vi "helper-snapshot-list.vi"(10 "ADDR":u8=1 min=1 max=99 step=1, 11 "IOnodes in":T1[](array[typedef])=[{"ADDR"=307, "Label"="ACID", "Type"=enum."DO", "Mode"=enum."RIO", "Value"="", "Tags"="", "calibration"=[{"X"=0.0, "Y"=0.0}, {"X"=0.0, "Y"=0.0}]}, {"ADDR"=309, "Label"="ALFA1", "Type"=enum."DO", "Mode"=enum."RIO", "Value"="", "Tags"="", "calibration"=[{"X"=0.0, "Y"=0.0}, {"X"=0.0, "Y"=0.0}]}, {"ADDR"=305, "Label"="BASE", "Type"=enum."DO", "Mode"=enum."RIO", "Value"="", "Tags"="", "calibration"=[{"X"=0.0, "Y"=0.0}, {"X"=0.0, "Y"=0.0}]}, {"ADDR"=311, "Label"="BETA1", "Type"=enum."DO", "Mode"=enum."RIO", "Value"="", "Tags"="", "calibration"=[{"X"=0.0, "Y"=0.0}, {"X"=0.0, "Y"=0.0}]}, {"ADDR"=210, "Label"="CIRCULATORS", "Type"=enum."DO", "Mode"=enum."RIO", "Value"="", "Tags"="", "calibration"=[{"X"=0.0, "Y"=0.0}, {"X"=0.0, "Y"=0.0}]}, {"ADDR"=200, "Label"="CNET", "Type"=enum."DO", "Mode"=enum."RIO", "Value"="", "Tags"="", "calibration"=[{"X"=0.0, "Y"=0.0}, {"X"=0.0, "Y"=0.0}]}, {"ADDR"=201, "Label"="CNETFOG", "Type"=enum."DO", "Mode"=enum."RIO", "Value"="", "Tags"="", "calibration"=[{"X"=0.0, "Y"=0.0}, {"X"=0.0, "Y"=0.0}]}, {"ADDR"=117, "Label"="CO2", "Type"=enum."DO", "Mode"=enum."RIO", "Value"="", "Tags"="", "calibration"=[{"X"=0.0, "Y"=0.0}, {"X"=0.0, "Y"=0.0}]}, {"ADDR"=316, "Label"="COLCHIL", "Type"=enum."DO", "Mode"=enum."RIO", "Value"="", "Tags"="", "calibration"=[{"X"=0.0, "Y"=0.0}, {"X"=0.0, "Y"=0.0}]}, {"ADDR"=112, "Label"="COOLFAN", "Type"=enum."DO", "Mode"=enum."RIO", "Value"="", "Tags"="", "calibration"=[{"X"=0.0, "Y"=0.0}, {"X"=0.0, "Y"=0.0}]}, {"ADDR"=211, "Label"="FECTORY_VENT", "Type"=enum."DO", "Mode"=enum."RIO", "Value"="", "Tags"="", "calibration"=[{"X"=0.0, "Y"=0.0}, {"X"=0.0, "Y"=0.0}]}, {"ADDR"=208, "Label"="H1_CURTAIN", "Type"=enum."DO", "Mode"=enum."RIO", "Value"="", "Tags"="", "calibration"=[{"X"=0.0, "Y"=0.0}, {"X"=0.0, "Y"=0.0}]}, {"ADDR"=215, "Label"="H1_FAN1", "Type"=enum."DO", "Mode"=enum."RIO", "Value"="", "Tags"="", "calibration"=[{"X"=0.0, "Y"=0.0}, {"X"=0.0, "Y"=0.0}]}, {"ADDR"=217, "Label"="H1_FAN2", "Type"=enum."DO", "Mode"=enum."RIO", "Value"="", "Tags"="", "calibration"=[{"X"=0.0, "Y"=0.0}, {"X"=0.0, "Y"=0.0}]}, {"ADDR"=209, "Label"="H1_FAN3", "Type"=enum."DO", "Mode"=enum."RIO", "Value"="", "Tags"="", "calibration"=[{"X"=0.0, "Y"=0.0}, {"X"=0.0, "Y"=0.0}]}, {"ADDR"=101, "Label"="H1_TDRY", "Type"=enum."AI", "Mode"=enum."RIO", "Value"="", "Tags"="", "calibration"=[{"X"=750.0, "Y"=18.0}, {"X"=1208.0, "Y"=25.0}]}, {"ADDR"=100, "Label"="H1_TWET", "Type"=enum."AI", "Mode"=enum."RIO", "Value"="", "Tags"="", "calibration"=[{"X"=800.0, "Y"=18.0}, {"X"=1500.0, "Y"=24.0}]}, {"ADDR"=205, "Label"="H1_WETPAD", "Type"=enum."DO", "Mode"=enum."RIO", "Value"="", "Tags"="", "calibration"=[{"X"=0.0, "Y"=0.0}, {"X"=0.0, "Y"=0.0}]}, {"ADDR"=205, "Label"="H2_TDRY", "Type"=enum."AI", "Mode"=enum."RIO", "Value"="", "Tags"="", "calibration"=[{"X"=600.0, "Y"=3.0}, {"X"=711.0, "Y"=23.0}]}, {"ADDR"=103, "Label"="H3_TDRY", "Type"=enum."AI", "Mode"=enum."RIO", "Value"="", "Tags"="", "calibration"=[{"X"=0.0, "Y"=0.0}, {"X"=0.0, "Y"=0.0}]}, {"ADDR"=105, "Label"="H3_TWET", "Type"=enum."AI", "Mode"=enum."RIO", "Value"="", "Tags"="", "calibration"=[{"X"=0.0, "Y"=0.0}, {"X"=0.0, "Y"=0.0}]}, {"ADDR"=400, "Label"="H4_TDRY", "Type"=enum."AI", "Mode"=enum."RIO", "Value"="", "Tags"="", "calibration"=[{"X"=0.0, "Y"=0.0}, {"X"=0.0, "Y"=0.0}]}, {"ADDR"=115, "Label"="IRR_NTR", "Type"=enum."DO", "Mode"=enum."RIO", "Value"="", "Tags"="", "calibration"=[{"X"=0.0, "Y"=0.0}, {"X"=0.0, "Y"=0.0}]}, {"ADDR"=315, "Label"="IRR_SEC1", "Type"=enum."DO", "Mode"=enum."RIO", "Value"="", "Tags"="", "calibration"=[{"X"=0.0, "Y"=0.0}, {"X"=0.0, "Y"=0.0}]}, {"ADDR"=606, "Label"="IRR_SEC2", "Type"=enum."DO", "Mode"=enum."RIO", "Value"="", "Tags"="", "calibration"=[{"X"=0.0, "Y"=0.0}, {"X"=0.0, "Y"=0.0}]}, {"ADDR"=212, "Label"="IRR_WTR", "Type"=enum."DO", "Mode"=enum."RIO", "Value"="", "Tags"="", "calibration"=[{"X"=0.0, "Y"=0.0}, {"X"=0.0, "Y"=0.0}]}, {"ADDR"=317, "Label"="MAINBLOWER", "Type"=enum."DO", "Mode"=enum."RIO", "Value"="", "Tags"="", "calibration"=[{"X"=0.0, "Y"=0.0}, {"X"=0.0, "Y"=0.0}]}, {"ADDR"=111, "Label"="NFTUP", "Type"=enum."DO", "Mode"=enum."RIO", "Value"="", "Tags"="", "calibration"=[{"X"=0.0, "Y"=0.0}, {"X"=0.0, "Y"=0.0}]}, {"ADDR"=306, "Label"="ORPMIX", "Type"=enum."DO", "Mode"=enum."RIO", "Value"="", "Tags"="", "calibration"=[{"X"=0.0, "Y"=0.0}, {"X"=0.0, "Y"=0.0}]}, {"ADDR"=510, "Label"="PBR_ABC_MEDIUM", "Type"=enum."DO", "Mode"=enum."RIO", "Value"="", "Tags"="", "calibration"=[{"X"=0.0, "Y"=0.0}, {"X"=0.0, "Y"=0.0}]}, {"ADDR"=525, "Label"="PBR_BIOM_LEVEL", "Type"=enum."DI", "Mode"=enum."RIO", "Value"="", "Tags"="", "calibration"=[{"X"=0.0, "Y"=0.0}, {"X"=0.0, "Y"=0.0}]}, {"ADDR"=416, "Label"="PBR_COOLNET", "Type"=enum."DO", "Mode"=enum."RIO", "Value"="", "Tags"="", "calibration"=[{"X"=0.0, "Y"=0.0}, {"X"=0.0, "Y"=0.0}]}, {"ADDR"=509, "Label"="PBR_DIGEST", "Type"=enum."DO", "Mode"=enum."RIO", "Value"="", "Tags"="", "calibration"=[{"X"=0.0, "Y"=0.0}, {"X"=0.0, "Y"=0.0}]}, {"ADDR"=411, "Label"="PBR_HARVEST", "Type"=enum."DO", "Mode"=enum."RIO", "Value"="", "Tags"="", "calibration"=[{"X"=0.0, "Y"=0.0}, {"X"=0.0, "Y"=0.0}]}, {"ADDR"=516, "Label"="PBR_HARVEST_BED", "Type"=enum."DO", "Mode"=enum."RIO", "Value"="", "Tags"="", "calibration"=[{"X"=0.0, "Y"=0.0}, {"X"=0.0, "Y"=0.0}]}, {"ADDR"=417, "Label"="PBR_MEDIUMTAPS", "Type"=enum."DO", "Mode"=enum."RIO", "Value"="", "Tags"="", "calibration"=[{"X"=0.0, "Y"=0.0}, {"X"=0.0, "Y"=0.0}]}, {"ADDR"=404, "Label"="PBR_OSWTR", "Type"=enum."DO", "Mode"=enum."RIO", "Value"="", "Tags"="", "calibration"=[{"X"=0.0, "Y"=0.0}, {"X"=0.0, "Y"=0.0}]}, {"ADDR"=514, "Label"="PBR_SANI", "Type"=enum."DO", "Mode"=enum."RIO", "Value"="", "Tags"="", "calibration"=[{"X"=0.0, "Y"=0.0}, {"X"=0.0, "Y"=0.0}]}, {"ADDR"=422, "Label"="PBR_SANI_RUN", "Type"=enum."DI", "Mode"=enum."RIO", "Value"="", "Tags"="", "calibration"=[{"X"=0.0, "Y"=0.0}, {"X"=0.0, "Y"=0.0}]}, {"ADDR"=513, "Label"="PBR_SNI_BED", "Type"=enum."DO", "Mode"=enum."RIO", "Value"="", "Tags"="", "calibration"=[{"X"=0.0, "Y"=0.0}, {"X"=0.0, "Y"=0.0}]}, {"ADDR"=511, "Label"="PBR_SNI_DRAIN", "Type"=enum."DO", "Mode"=enum."RIO", "Value"="", "Tags"="", "calibration"=[{"X"=0.0, "Y"=0.0}, {"X"=0.0, "Y"=0.0}]}, {"ADDR"=512, "Label"="PBR_SNI_SINK", "Type"=enum."DO", "Mode"=enum."RIO", "Value"="", "Tags"="", "calibration"=[{"X"=0.0, "Y"=0.0}, {"X"=0.0, "Y"=0.0}]}, {"ADDR"=420, "Label"="PBR_SPARE_LEVEL", "Type"=enum."DI", "Mode"=enum."RIO", "Value"="", "Tags"="", "calibration"=[{"X"=0.0, "Y"=0.0}, {"X"=0.0, "Y"=0.0}]}, {"ADDR"=0, "Label"="PBR_T1", "Type"=enum."AI", "Mode"=enum."RIO", "Value"="", "Tags"="", "calibration"=[{"X"=705.0, "Y"=21.0}, {"X"=1275.0, "Y"=36.4}]}, {"ADDR"=0, "Label"="PBR_T2", "Type"=enum."AI", "Mode"=enum."RIO", "Value"="", "Tags"="", "calibration"=[{"X"=700.0, "Y"=21.0}, {"X"=950.0, "Y"=35.0}]}, {"ADDR"=415, "Label"="PBR_TAPWATER", "Type"=enum."DO", "Mode"=enum."RIO", "Value"="", "Tags"="", "calibration"=[{"X"=0.0, "Y"=0.0}, {"X"=0.0, "Y"=0.0}]}, {"ADDR"=402, "Label"="PBR_U1_COLLIN", "Type"=enum."DO", "Mode"=enum."RIO", "Value"="", "Tags"="", "calibration"=[{"X"=0.0, "Y"=0.0}, {"X"=0.0, "Y"=0.0}]}, {"ADDR"=403, "Label"="PBR_U1_COLLOUT", "Type"=enum."DO", "Mode"=enum."RIO", "Value"="", "Tags"="", "calibration"=[{"X"=0.0, "Y"=0.0}, {"X"=0.0, "Y"=0.0}]}, {"ADDR"=424, "Label"="PBR_U1_FLOW", "Type"=enum."DI", "Mode"=enum."RIO", "Value"="", "Tags"="", "calibration"=[{"X"=0.0, "Y"=0.0}, {"X"=0.0, "Y"=0.0}]}, {"ADDR"=409, "Label"="PBR_U1_MAIN", "Type"=enum."DO", "Mode"=enum."RIO", "Value"="", "Tags"="", "calibration"=[{"X"=0.0, "Y"=0.0}, {"X"=0.0, "Y"=0.0}]}, {"ADDR"=412, "Label"="PBR_U1_PUMP", "Type"=enum."DO", "Mode"=enum."RIO", "Value"="", "Tags"="", "calibration"=[{"X"=0.0, "Y"=0.0}, {"X"=0.0, "Y"=0.0}]}, {"ADDR"=410, "Label"="PBR_U1_TANKIN", "Type"=enum."DO", "Mode"=enum."RIO", "Value"="", "Tags"="", "calibration"=[{"X"=0.0, "Y"=0.0}, {"X"=0.0, "Y"=0.0}]}, {"ADDR"=400, "Label"="PBR_U1_TANKOUT", "Type"=enum."DO", "Mode"=enum."RIO", "Value"="", "Tags"="", "calibration"=[{"X"=0.0, "Y"=0.0}, {"X"=0.0, "Y"=0.0}]}, {"ADDR"=406, "Label"="PBR_U2_MAIN", "Type"=enum."DO", "Mode"=enum."RIO", "Value"="", "Tags"="", "calibration"=[{"X"=0.0, "Y"=0.0}, {"X"=0.0, "Y"=0.0}]}, {"ADDR"=515, "Label"="PBR_U2_PUMP", "Type"=enum."DO", "Mode"=enum."RIO", "Value"="", "Tags"="", "calibration"=[{"X"=0.0, "Y"=0.0}, {"X"=0.0, "Y"=0.0}]}, {"ADDR"=407, "Label"="PBR_U3_COLLIN", "Type"=enum."DO", "Mode"=enum."RIO", "Value"="", "Tags"="", "calibration"=[{"X"=0.0, "Y"=0.0}, {"X"=0.0, "Y"=0.0}]}, {"ADDR"=408, "Label"="PBR_U3_COLLOUT", "Type"=enum."DO", "Mode"=enum."RIO", "Value"="", "Tags"="", "calibration"=[{"X"=0.0, "Y"=0.0}, {"X"=0.0, "Y"=0.0}]}, {"ADDR"=425, "Label"="PBR_U3_FLOW", "Type"=enum."DI", "Mode"=enum."RIO", "Value"="", "Tags"="", "calibration"=[{"X"=0.0, "Y"=0.0}, {"X"=0.0, "Y"=0.0}]}, {"ADDR"=401, "Label"="PBR_U3_MAIN", "Type"=enum."DO", "Mode"=enum."RIO", "Value"="", "Tags"="", "calibration"=[{"X"=0.0, "Y"=0.0}, {"X"=0.0, "Y"=0.0}]}, {"ADDR"=413, "Label"="PBR_U3_PUMP", "Type"=enum."DO", "Mode"=enum."RIO", "Value"="", "Tags"="", "calibration"=[{"X"=0.0, "Y"=0.0}, {"X"=0.0, "Y"=0.0}]}, {"ADDR"=405, "Label"="PBR_U3_TANKIN", "Type"=enum."DO", "Mode"=enum."RIO", "Value"="", "Tags"="", "calibration"=[{"X"=0.0, "Y"=0.0}, {"X"=0.0, "Y"=0.0}]}, {"ADDR"=414, "Label"="PBR_U3_TANKOUT", "Type"=enum."DO", "Mode"=enum."RIO", "Value"="", "Tags"="", "calibration"=[{"X"=0.0, "Y"=0.0}, {"X"=0.0, "Y"=0.0}]}, {"ADDR"=118, "Label"="RFSSW_1", "Type"=enum."DI", "Mode"=enum."RIO", "Value"="", "Tags"="", "calibration"=[{"X"=0.0, "Y"=0.0}, {"X"=0.0, "Y"=0.0}]}, {"ADDR"=119, "Label"="RFSSW_2", "Type"=enum."DI", "Mode"=enum."RIO", "Value"="", "Tags"="", "calibration"=[{"X"=0.0, "Y"=0.0}, {"X"=0.0, "Y"=0.0}]}, {"ADDR"=133, "Label"="RFSSW_3", "Type"=enum."DI", "Mode"=enum."RIO", "Value"="", "Tags"="", "calibration"=[{"X"=0.0, "Y"=0.0}, {"X"=0.0, "Y"=0.0}]}, {"ADDR"=144, "Label"="RFSSW_4", "Type"=enum."DI", "Mode"=enum."RIO", "Value"="", "Tags"="", "calibration"=[{"X"=0.0, "Y"=0.0}, {"X"=0.0, "Y"=0.0}]}, {"ADDR"=143, "Label"="RFSSW_5", "Type"=enum."DI", "Mode"=enum."RIO", "Value"="", "Tags"="", "calibration"=[{"X"=0.0, "Y"=0.0}, {"X"=0.0, "Y"=0.0}]}, {"ADDR"=201, "Label"="RFSX1", "Type"=enum."DO", "Mode"=enum."RIO", "Value"="", "Tags"="", "calibration"=[{"X"=0.0, "Y"=0.0}, {"X"=0.0, "Y"=0.0}]}, {"ADDR"=203, "Label"="RFSX2", "Type"=enum."DO", "Mode"=enum."RIO", "Value"="", "Tags"="", "calibration"=[{"X"=0.0, "Y"=0.0}, {"X"=0.0, "Y"=0.0}]}, {"ADDR"=107, "Label"="RFSX4", "Type"=enum."DO", "Mode"=enum."RIO", "Value"="", "Tags"="", "calibration"=[{"X"=0.0, "Y"=0.0}, {"X"=0.0, "Y"=0.0}]}, {"ADDR"=100, "Label"="RFSY1", "Type"=enum."DO", "Mode"=enum."RIO", "Value"="", "Tags"="", "calibration"=[{"X"=0.0, "Y"=0.0}, {"X"=0.0, "Y"=0.0}]}, {"ADDR"=102, "Label"="RFSY2", "Type"=enum."DO", "Mode"=enum."RIO", "Value"="", "Tags"="", "calibration"=[{"X"=0.0, "Y"=0.0}, {"X"=0.0, "Y"=0.0}]}, {"ADDR"=216, "Label"="STIRER", "Type"=enum."DO", "Mode"=enum."RIO", "Value"="", "Tags"="", "calibration"=[{"X"=0.0, "Y"=0.0}, {"X"=0.0, "Y"=0.0}]}, {"ADDR"=203, "Label"="TDRY", "Type"=enum."AI", "Mode"=enum."RIO", "Value"="", "Tags"="", "calibration"=[{"X"=1600.0, "Y"=1.0}, {"X"=1800.0, "Y"=22.0}]}, {"ADDR"=202, "Label"="TWET", "Type"=enum."AI", "Mode"=enum."RIO", "Value"="", "Tags"="", "calibration"=[{"X"=700.0, "Y"=0.4}, {"X"=1800.0, "Y"=23.0}]}, {"ADDR"=301, "Label"="UN_EC", "Type"=enum."AI", "Mode"=enum."RIO", "Value"="", "Tags"="", "calibration"=[{"X"=878.0, "Y"=0.0}, {"X"=955.0, "Y"=1.5}]}, {"ADDR"=302, "Label"="UN_ORP", "Type"=enum."AI", "Mode"=enum."RIO", "Value"="", "Tags"="", "calibration"=[{"X"=33.0, "Y"=0.0}, {"X"=902.0, "Y"=329.0}]}, {"ADDR"=300, "Label"="UN_PH", "Type"=enum."AI", "Mode"=enum."RIO", "Value"="", "Tags"="", "calibration"=[{"X"=600.0, "Y"=0.0}, {"X"=1800.0, "Y"=6.59}]}, {"ADDR"=304, "Label"="UN_PH2", "Type"=enum."AI", "Mode"=enum."RIO", "Value"="", "Tags"="", "calibration"=[{"X"=100.0, "Y"=4.0}, {"X"=636.0, "Y"=6.6}]}, {"ADDR"=113, "Label"="UN_PMP1", "Type"=enum."DO", "Mode"=enum."RIO", "Value"="", "Tags"="", "calibration"=[{"X"=0.0, "Y"=0.0}, {"X"=0.0, "Y"=0.0}]}, {"ADDR"=114, "Label"="UN_PMP2", "Type"=enum."DO", "Mode"=enum."RIO", "Value"="", "Tags"="", "calibration"=[{"X"=0.0, "Y"=0.0}, {"X"=0.0, "Y"=0.0}]}, {"ADDR"=110, "Label"="UN_PMP3", "Type"=enum."DO", "Mode"=enum."RIO", "Value"="", "Tags"="", "calibration"=[{"X"=0.0, "Y"=0.0}, {"X"=0.0, "Y"=0.0}]}, {"ADDR"=301, "Label"="UN_PMP4", "Type"=enum."DO", "Mode"=enum."RIO", "Value"="", "Tags"="", "calibration"=[{"X"=0.0, "Y"=0.0}, {"X"=0.0, "Y"=0.0}]}, {"ADDR"=116, "Label"="UN_PMP5", "Type"=enum."DO", "Mode"=enum."RIO", "Value"="", "Tags"="", "calibration"=[{"X"=0.0, "Y"=0.0}, {"X"=0.0, "Y"=0.0}]}, {"ADDR"=213, "Label"="UN_VLV1", "Type"=enum."DO", "Mode"=enum."RIO", "Value"="", "Tags"="", "calibration"=[{"X"=0.0, "Y"=0.0}, {"X"=0.0, "Y"=0.0}]}, {"ADDR"=310, "Label"="UN_VLV2", "Type"=enum."DO", "Mode"=enum."RIO", "Value"="", "Tags"="", "calibration"=[{"X"=0.0, "Y"=0.0}, {"X"=0.0, "Y"=0.0}]}, {"ADDR"=312, "Label"="UN_VLV3", "Type"=enum."DO", "Mode"=enum."RIO", "Value"="", "Tags"="", "calibration"=[{"X"=0.0, "Y"=0.0}, {"X"=0.0, "Y"=0.0}]}, {"ADDR"=308, "Label"="UN_VLV5", "Type"=enum."DO", "Mode"=enum."RIO", "Value"="", "Tags"="", "calibration"=[{"X"=0.0, "Y"=0.0}, {"X"=0.0, "Y"=0.0}]}, {"ADDR"=123, "Label"="UN_WL1", "Type"=enum."DI", "Mode"=enum."RIO", "Value"="", "Tags"="", "calibration"=[{"X"=0.0, "Y"=0.0}, {"X"=0.0, "Y"=0.0}]}, {"ADDR"=125, "Label"="UN_WL2", "Type"=enum."DI", "Mode"=enum."RIO", "Value"="", "Tags"="", "calibration"=[{"X"=0.0, "Y"=0.0}, {"X"=0.0, "Y"=0.0}]}, {"ADDR"=124, "Label"="UN_WL3", "Type"=enum."DI", "Mode"=enum."RIO", "Value"="", "Tags"="", "calibration"=[{"X"=0.0, "Y"=0.0}, {"X"=0.0, "Y"=0.0}]}, {"ADDR"=136, "Label"="UN_WL4", "Type"=enum."DI", "Mode"=enum."RIO", "Value"="", "Tags"="", "calibration"=[{"X"=0.0, "Y"=0.0}, {"X"=0.0, "Y"=0.0}]}, {"ADDR"=121, "Label"="UN_WL5", "Type"=enum."DI", "Mode"=enum."RIO", "Value"="", "Tags"="", "calibration"=[{"X"=0.0, "Y"=0.0}, {"X"=0.0, "Y"=0.0}]}, {"ADDR"=303, "Label"="UN_WT", "Type"=enum."AI", "Mode"=enum."RIO", "Value"="", "Tags"="", "calibration"=[{"X"=120.0, "Y"=16.0}, {"X"=626.0, "Y"=28.0}]}, {"ADDR"=102, "Label"="UV", "Type"=enum."AI", "Mode"=enum."RIO", "Value"="", "Tags"="", "calibration"=[{"X"=493.0, "Y"=0.0}, {"X"=1071.0, "Y"=650.0}]}, {"ADDR"=314, "Label"="WATER", "Type"=enum."DO", "Mode"=enum."RIO", "Value"="", "Tags"="", "calibration"=[{"X"=0.0, "Y"=0.0}, {"X"=0.0, "Y"=0.0}]}, {"ADDR"=214, "Label"="WETWALL", "Type"=enum."DO", "Mode"=enum."RIO", "Value"="", "Tags"="", "calibration"=[{"X"=0.0, "Y"=0.0}, {"X"=0.0, "Y"=0.0}]}, {"ADDR"=200, "Label"="W_DIR", "Type"=enum."AI", "Mode"=enum."RIO", "Value"="", "Tags"="", "calibration"=[{"X"=0.0, "Y"=0.0}, {"X"=4000.0, "Y"=360.0}]}, {"ADDR"=201, "Label"="W_SPD", "Type"=enum."AI", "Mode"=enum."RIO", "Value"="", "Tags"="", "calibration"=[{"X"=0.0, "Y"=1.0}, {"X"=4000.0, "Y"=100.0}]}] {"calibration"."Y" format="%#.3f"; "calibration"."X" format="%#.3f"; "ADDR" format="%04d"}) -> (3 "IOcon snapshot list out":T1[](array[typedef]) {"calibration"."Y" format="%#.3f"; "calibration"."X" format="%#.3f"; "ADDR" format="%04d"})   [LabVIEW 2024]
uses:
  controls/IONode.ctl
  controls/type.address.ctl
  controls/enum.io.type.ctl
  controls/enum.io.mode.ctl
  controls/typeXyPoint.ctl
  controls/enumVarCtrlIO.ctl
  controls/enum-io-sort-type.ctl
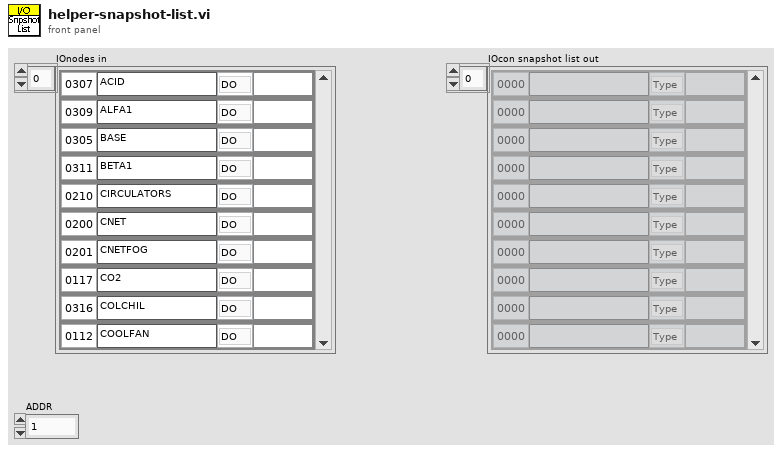
[diagram p1: front panel]
types:
  T1 = typedef "IONode.ctl" = cluster{"ADDR":T2, "Label":string, "Type":T3, "Mode":T4, "Value":string, "Tags":string, "calibration":T5[]}
  T2 = typedef "type.address.ctl" = u16
  T3 = typedef "enum.io.type.ctl" = enum16{"Type", "DI", "DO", "AI", "AO", "VL", "BUF"}
  T4 = typedef "enum.io.mode.ctl" = enum16{"Mode", "RIO", "SIM"}
  T5 = typedef "typeXyPoint.ctl" = cluster{"X":dbl, "Y":dbl}
  T6 = cluster{"ADDR":u8, "Label":string, "Type":T3, "Mode":T4, "Tags":string}
  T7 = typedef "enumVarCtrlIO.ctl" = enum16{"IO Get By Key", "IO List Configs", "IO Add By Key", "IO Modify Value By Key", "IO Modify Calib By Key", "IO Modify ADDR By Key", "IO Modify Mode By Key", "IO Modify Type By Key", "IO Modify Name By Key", "IO Remove By Key", "IO Remove All"}
  T8 = typedef "enum-io-sort-type.ctl" = enum16{"Sort By Address", "Sort By Name"}
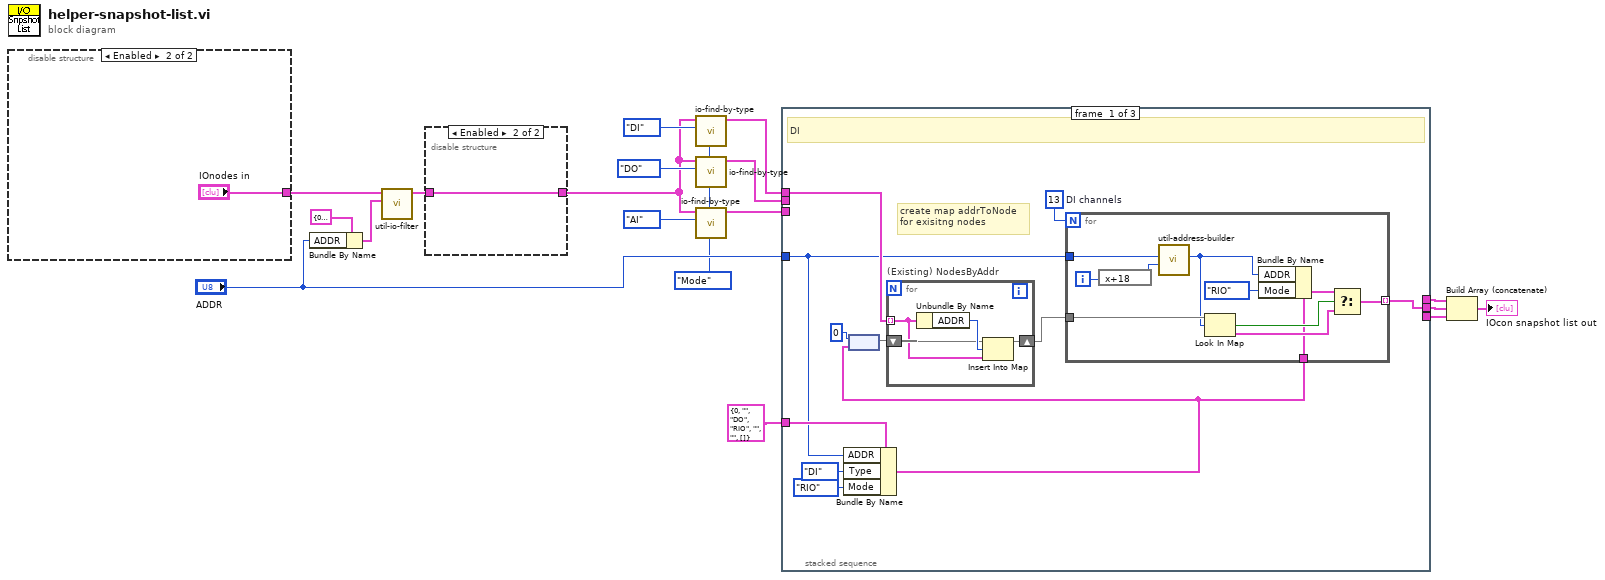
[diagram p0: block diagram]
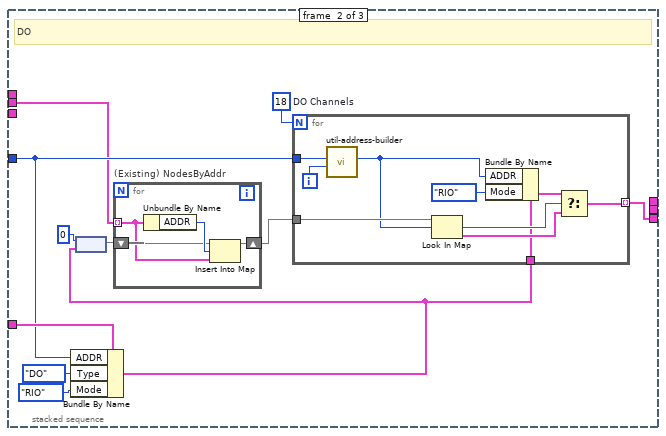
[diagram p2: hidden frame]
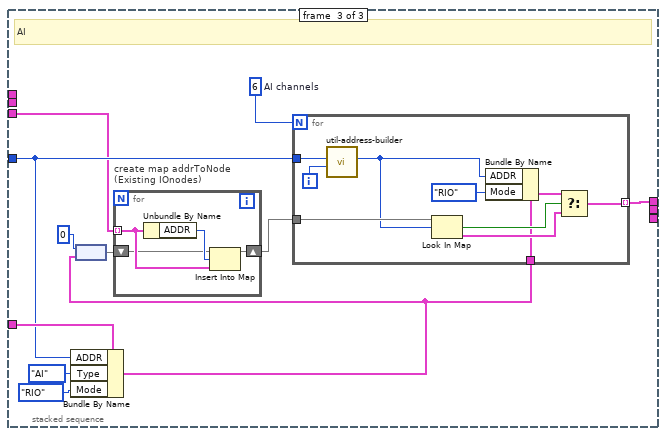
[diagram p3: hidden frame]
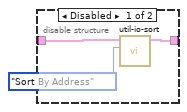
[diagram p4: hidden frame]
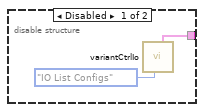
[diagram p5: hidden frame]
diagram:
  w6 = enum.io.mode."Mode" ("Mode(Any)")
  n1 = disable-structure shown="Enabled" {
    disable-tunnel: [w20 "IOnodes in"] -> w18
    frame Disabled {
      n2 = call "variantCtrlIo.vi"("menu (Get Param)"=enumVarCtrlIO."IO List Configs") -> ("IO Configs List"=w20:T1[])  [unwired: 6 in, 4 out]
    }
    frame Enabled {
    }
  }
  n3 = Bundle By Name(cluster=T6 {"ADDR"=0, "Label"="", "Type"=enum."Type", "Mode"=enum."Mode", "Tags"=""} ("IO Search Conf"), "ADDR"="ADDR") -> (w16:T6)
  n4 = call "util-io-filter.vi"("IO Search Conf"=w16, "IO Configs List"=w18) -> ("Search Results"=w17:T1[])  [unwired: 9 in]
  n5 = disable-structure shown="Enabled" {
    disable-tunnel: w17 -> [w24 w25]
    disable-tunnel: [w23 w25] -> w10
    frame Disabled {
      n6 = call "util-io-sort.vi"(10:enum-io-sort-type."Sort By Address", "IO Configs List"=w24) -> ("Result"=w23:T1[])  [unwired: 9 in]
    }
    frame Enabled {
    }
  }
  n7 = call "io-find-by-type.vi"("Mode(Any)"=w6, "Type"=enum.io.type."DI", "IOConfigs in"=w10) -> ("Search Results"=w7:T1[])  [unwired: 8 in]
  n8 = call "io-find-by-type.vi"("Mode(Any)"=w6, "Type"=enum.io.type."DO", "IOConfigs in"=w10) -> ("Search Results"=w8:T1[])  [unwired: 8 in]
  n9 = call "io-find-by-type.vi"("Mode(Any)"=w6, "Type"=enum.io.type."AI", "IOConfigs in"=w10) -> ("Search Results"=w9:T1[])  [unwired: 8 in]
  n10 = stacked-sequence {
    tunnel: "ADDR" -> [w28 w56 w81]
    tunnel: w8 -> [_ w52 _]
    tunnel: [_ w54 _] -> w3
    tunnel: w7 -> [w32 _ _]
    tunnel: [w31 _ _] -> w2
    tunnel: w9 -> [_ _ w77]
    tunnel: T1 {"ADDR"=0, "Label"="", "Type"=enum."DO", "Mode"=enum."RIO", "Value"="", "Tags"="", "calibration"=[]} ("Search Results") -> [w29 w57 w82]
    tunnel: [_ _ w78] -> w1
    frame #0 {
      w36 = 13  # DI channels
      # "create map addrToNode\nfor exisitng nodes"
      # "DI"
      n11 = Bundle By Name(cluster=w29, "ADDR"=w28, "Type"=enum.io.type."DI", "Mode"=enum.io.mode."RIO") -> (w30:T1)
      n12 = node(T2 0 ("ADDR"), w30) -> (w35:map{T2, T1})
      n13 = for "(Existing) NodesByAddr" {
        tunnel: w32 -> [w39] mode=indexing
        shift-right: [w38] -> w33
        shift-left: w35 -> [w37]
        n14 = Unbundle By Name(w39) -> ("ADDR"=w40:T2)
        n15 = Insert Into Map(map in=w37, key=w40, value=w39) -> (map out=w38:map{T2, T1})  [unwired: 2 out]
      }
      n16 = for {
        N: w36 -> [_]
        tunnel: w28 -> [w50]
        tunnel: w33 -> [w49]
        tunnel: [w46] -> w31 mode=indexing
        tunnel: w30 -> [w42]
        i -> [w51]
        n17 = expression code="x+18"(w51) -> (w41:i32)
        n18 = call "util-address-builder.vi"("Channel"=w41, "Device"=w50) -> ("ADDR"=w44:T2)  [unwired: 9 in]
        n19 = Look In Map(map=w49, key=w44) -> (key not found?=w48:bool, value=w47:T1)  [unwired: 1 in]
        n20 = Bundle By Name(cluster=w42, "ADDR"=w44, "Mode"=enum.io.mode."RIO") -> (w45:T1)
        n21 = Select(t=w45, s=w48, f=w47) -> (s? t:f=w46:T1)
      }
    }
    frame #1 {
      w62 = 18  # DO Channels
      # "DO"
      n22 = Bundle By Name(cluster=w57, "ADDR"=w56, "Type"=enum.io.type."DO", "Mode"=enum.io.mode."RIO") -> (w58:T1)
      n23 = node(T2 0 ("ADDR"), w58) -> (w61:map{T2, T1})
      n24 = for "(Existing) NodesByAddr" {
        tunnel: w52 -> [w65] mode=indexing
        shift-right: [w64] -> w59
        shift-left: w61 -> [w63]
        n25 = Unbundle By Name(w65) -> ("ADDR"=w66:T2)
        n26 = Insert Into Map(map in=w63, key=w66, value=w65) -> (map out=w64:map{T2, T1})  [unwired: 2 out]
      }
      n27 = for {
        N: w62 -> [_]
        tunnel: w56 -> [w75]
        tunnel: w59 -> [w74]
        tunnel: [w71] -> w54 mode=indexing
        tunnel: w58 -> [w67]
        i -> [w76]
        n28 = call "util-address-builder.vi"("Channel"=w76, "Device"=w75) -> ("ADDR"=w69:T2)  [unwired: 9 in]
        n29 = Look In Map(map=w74, key=w69) -> (key not found?=w73:bool, value=w72:T1)  [unwired: 1 in]
        n30 = Bundle By Name(cluster=w67, "ADDR"=w69, "Mode"=enum.io.mode."RIO") -> (w70:T1)
        n31 = Select(t=w70, s=w73, f=w72) -> (s? t:f=w71:T1)
      }
    }
    frame #2 {
      w87 = 6  # AI channels
      # "AI"
      n32 = Bundle By Name(cluster=w82, "ADDR"=w81, "Type"=enum.io.type."AI", "Mode"=enum.io.mode."RIO") -> (w83:T1)
      n33 = node(T2 0 ("ADDR"), w83) -> (w86:map{T2, T1})
      n34 = for "create map addrToNode\n(Existing IOnodes)" {
        tunnel: w77 -> [w90] mode=indexing
        shift-right: [w89] -> w84
        shift-left: w86 -> [w88]
        n35 = Unbundle By Name(w90) -> ("ADDR"=w91:T2)
        n36 = Insert Into Map(map in=w88, key=w91, value=w90) -> (map out=w89:map{T2, T1})  [unwired: 2 out]
      }
      n37 = for {
        N: w87 -> [_]
        tunnel: w81 -> [w100]
        tunnel: w84 -> [w99]
        tunnel: [w96] -> w78 mode=indexing
        tunnel: w83 -> [w92]
        i -> [w101]
        n38 = call "util-address-builder.vi"("Channel"=w101, "Device"=w100) -> ("ADDR"=w94:T2)  [unwired: 9 in]
        n39 = Look In Map(map=w99, key=w94) -> (key not found?=w98:bool, value=w97:T1)  [unwired: 1 in]
        n40 = Bundle By Name(cluster=w92, "ADDR"=w94, "Mode"=enum.io.mode."RIO") -> (w95:T1)
        n41 = Select(t=w95, s=w98, f=w97) -> (s? t:f=w96:T1)
      }
    }
  }
  n42 = Build Array (concatenate)(w1, w2, w3) -> (→"IOcon snapshot list out":T1[])
